vi "TalonFXConfigurator.vi"(6 "timeoutSeconds":dbl=0.05, 8 "error in":errorcluster, 10 "DeviceConfiguration":T2={"Future Proof Configs"=FALSE, "MotorOutputInverted"=0, "MotorOutputNeutralMode"=0, "MotorOutputDutyCycleNeutralDeadband"=0.0, "MotorOutputPeakForwardDutyCycle"=1.0, "MotorOutputPeakReverseDutyCycle"=-1.0, "CurrentLimitsStatorCurrentLimit"=0.0, "CurrentLimitsStatorCurrentLimitEnable"=FALSE, "CurrentLimitsSupplyCurrentLimit"=0.0, "CurrentLimitsSupplyCurrentLimitEnable"=FALSE, "CurrentLimitsSupplyCurrentThreshold"=0.0, "CurrentLimitsSupplyTimeThreshold"=0.0, "VoltageSupplyVoltageTimeConstant"=0.0, "VoltagePeakForwardVoltage"=16.0, "VoltagePeakReverseVoltage"=-16.0, "TorqueCurrentPeakForwardTorqueCurrent"=800.0, "TorqueCurrentPeakReverseTorqueCurrent"=-800.0, "TorqueCurrentTorqueNeutralDeadband"=0.0, "FeedbackFeedbackRotorOffset"=0.0, "FeedbackSensorToMechanismRatio"=1.0, "FeedbackRotorToSensorRatio"=1.0, "FeedbackFeedbackSensorSource"=0, "FeedbackFeedbackRemoteSensorID"=0, "DifferentialSensorsDifferentialSensorSource"=0, "DifferentialSensorsDifferentialTalonFXSensorID"=0, "DifferentialSensorsDifferentialRemoteSensorID"=0, "DifferentialConstantsPeakDifferentialDutyCycle"=2.0, "DifferentialConstantsPeakDifferentialVoltage"=32.0, "DifferentialConstantsPeakDifferentialTorqueCurrent"=1600.0, "OpenLoopRampsDutyCycleOpenLoopRampPeriod"=0.0, "OpenLoopRampsVoltageOpenLoopRampPeriod"=0.0, "OpenLoopRampsTorqueOpenLoopRampPeriod"=0.0, "ClosedLoopRampsDutyCycleClosedLoopRampPeriod"=0.0, "ClosedLoopRampsVoltageClosedLoopRampPeriod"=0.0, "ClosedLoopRampsTorqueClosedLoopRampPeriod"=0.0, "HardwareLimitSwitchForwardLimitType"=0, "HardwareLimitSwitchForwardLimitAutosetPositionEnable"=FALSE, "HardwareLimitSwitchForwardLimitAutosetPositionValue"=0.0, "HardwareLimitSwitchForwardLimitEnable"=TRUE, "HardwareLimitSwitchForwardLimitSource"=0, "HardwareLimitSwitchForwardLimitRemoteSensorID"=0, "HardwareLimitSwitchReverseLimitType"=0, "HardwareLimitSwitchReverseLimitAutosetPositionEnable"=FALSE, "HardwareLimitSwitchReverseLimitAutosetPositionValue"=0.0, "HardwareLimitSwitchReverseLimitEnable"=TRUE, "HardwareLimitSwitchReverseLimitSource"=0, "HardwareLimitSwitchReverseLimitRemoteSensorID"=0, "AudioBeepOnBoot"=TRUE, "AudioBeepOnConfig"=TRUE, "AudioAllowMusicDurDisable"=FALSE, "SoftwareLimitSwitchForwardSoftLimitEnable"=FALSE, "SoftwareLimitSwitchReverseSoftLimitEnable"=FALSE, "SoftwareLimitSwitchForwardSoftLimitThreshold"=0.0, "SoftwareLimitSwitchReverseSoftLimitThreshold"=0.0, "MotionMagicMotionMagicCruiseVelocity"=0.0, "MotionMagicMotionMagicAcceleration"=0.0, "MotionMagicMotionMagicJerk"=0.0, "MotionMagicMotionMagicExpo_kV"=0.0, "MotionMagicMotionMagicExpo_kA"=0.0, "CustomParamsCustomParam0"=0, "CustomParamsCustomParam1"=0, "ClosedLoopGeneralContinuousWrap"=FALSE, "Slot0kP"=0.0, "Slot0kI"=0.0, "Slot0kD"=0.0, "Slot0kS"=0.0, "Slot0kV"=0.0, "Slot0kA"=0.0, "Slot0kG"=0.0, "Slot0GravityType"=0, "Slot0StaticFeedforwardSign"=0, "Slot1kP"=0.0, "Slot1kI"=0.0, "Slot1kD"=0.0, "Slot1kS"=0.0, "Slot1kV"=0.0, "Slot1kA"=0.0, "Slot1kG"=0.0, "Slot1GravityType"=0, "Slot1StaticFeedforwardSign"=0, "Slot2kP"=0.0, "Slot2kI"=0.0, "Slot2kD"=0.0, "Slot2kS"=0.0, "Slot2kV"=0.0, "Slot2kA"=0.0, "Slot2kG"=0.0, "Slot2GravityType"=0, "Slot2StaticFeedforwardSign"=0} {"MotorOutputInverted" items=["CounterClockwise_Positive", "Clockwise_Positive"]; "MotorOutputNeutralMode" items=["Coast", "Brake"]; "FeedbackFeedbackSensorSource" items=["RotorSensor", "RemoteCANcoder", "RemotePigeon2_Yaw", "RemotePigeon2_Pitch", "RemotePigeon2_Roll", "FusedCANcoder", "SyncCANcoder"]; "DifferentialSensorsDifferentialSensorSource" items=["Disabled", "RemoteTalonFX_Diff", "RemotePigeon2_Yaw", "RemotePigeon2_Pitch", "RemotePigeon2_Roll", "RemoteCANcoder"]; "HardwareLimitSwitchForwardLimitType" items=["NormallyOpen", "NormallyClosed"]; "HardwareLimitSwitchForwardLimitSource" items=["LimitSwitchPin"=0, "RemoteTalonFX"=1, "RemoteCANifier"=2, "RemoteCANcoder"=4, "Disabled"=3]; "HardwareLimitSwitchReverseLimitType" items=["NormallyOpen", "NormallyClosed"]; "HardwareLimitSwitchReverseLimitSource" items=["LimitSwitchPin"=0, "RemoteTalonFX"=1, "RemoteCANifier"=2, "RemoteCANcoder"=4, "Disabled"=3]; "Slot0GravityType" items=["Elevator_Static", "Arm_Cosine"]; "Slot0StaticFeedforwardSign" items=["UseVelocitySign", "UseClosedLoopSign"]; "Slot1GravityType" items=["Elevator_Static", "Arm_Cosine"]; "Slot1StaticFeedforwardSign" items=["UseVelocitySign", "UseClosedLoopSign"]; "Slot2GravityType" items=["Elevator_Static", "Arm_Cosine"]; "Slot2StaticFeedforwardSign" items=["UseVelocitySign", "UseClosedLoopSign"]}, 11 "DeviceReference":T1) -> (0 "error out":errorcluster)   [LabVIEW 2023]
uses:
  Users/Cory/Documents/PhoenixPro-LabVIEW-Generation/controls/DeviceReference.ctl
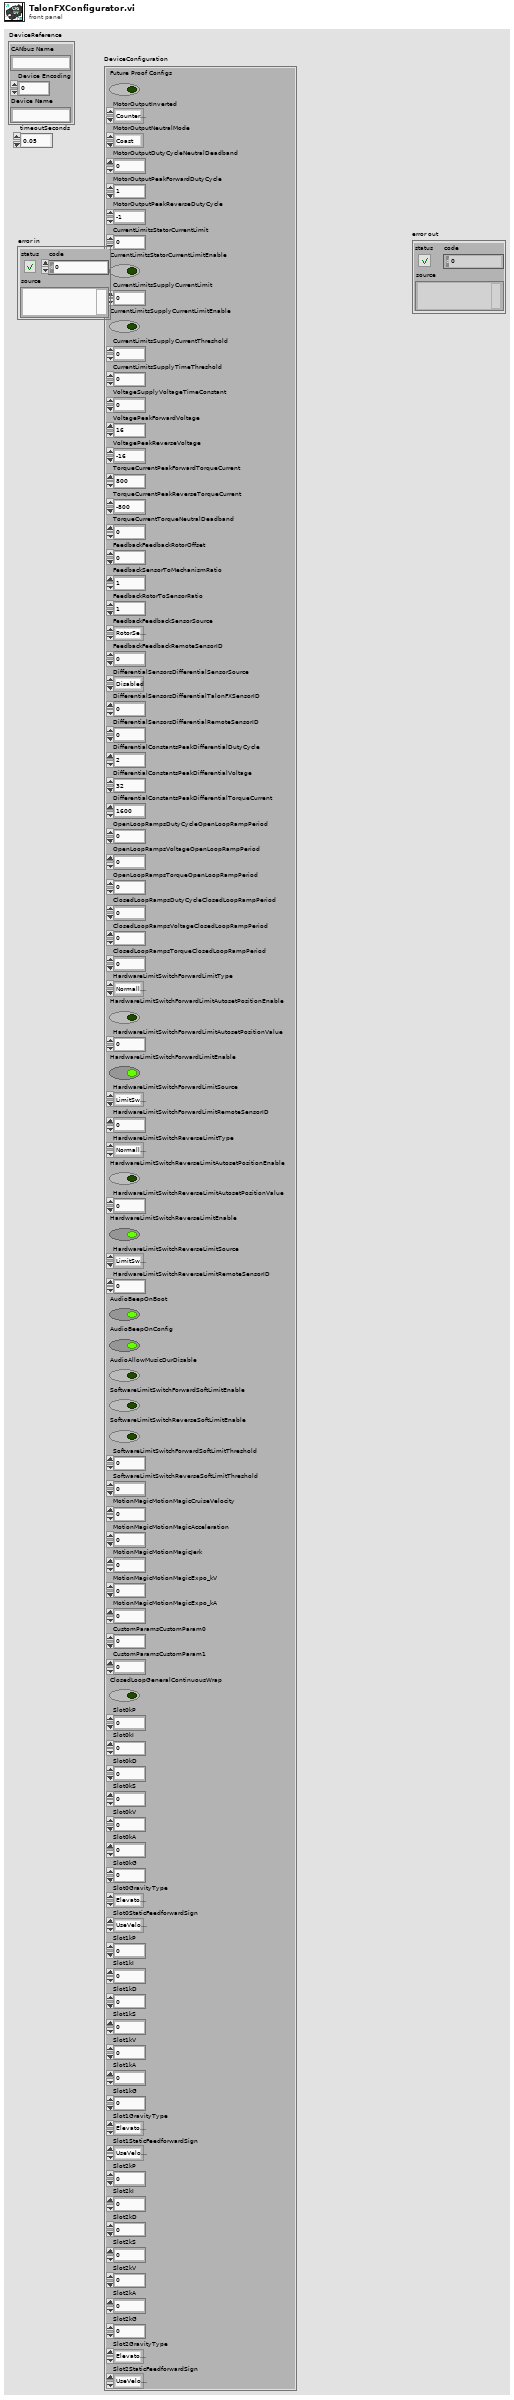
[diagram p1: front panel]
types:
  T1 = typedef "DeviceReference.ctl" = cluster{"CANbus Name":string, "Device Encoding":u32, "Device Name":string}
  T2 = cluster{"Future Proof Configs":bool, "MotorOutputInverted":u16, "MotorOutputNeutralMode":u16, "MotorOutputDutyCycleNeutralDeadband":dbl, "MotorOutputPeakForwardDutyCycle":dbl, "MotorOutputPeakReverseDutyCycle":dbl, "CurrentLimitsStatorCurrentLimit":dbl, "CurrentLimitsStatorCurrentLimitEnable":bool, "CurrentLimitsSupplyCurrentLimit":dbl, "CurrentLimitsSupplyCurrentLimitEnable":bool, "CurrentLimitsSupplyCurrentThreshold":dbl, "CurrentLimitsSupplyTimeThreshold":dbl, "VoltageSupplyVoltageTimeConstant":dbl, "VoltagePeakForwardVoltage":dbl, "VoltagePeakReverseVoltage":dbl, "TorqueCurrentPeakForwardTorqueCurrent":dbl, "TorqueCurrentPeakReverseTorqueCurrent":dbl, "TorqueCurrentTorqueNeutralDeadband":dbl, "FeedbackFeedbackRotorOffset":dbl, "FeedbackSensorToMechanismRatio":dbl, "FeedbackRotorToSensorRatio":dbl, "FeedbackFeedbackSensorSource":u16, "FeedbackFeedbackRemoteSensorID":i16, "DifferentialSensorsDifferentialSensorSource":u16, "DifferentialSensorsDifferentialTalonFXSensorID":i16, "DifferentialSensorsDifferentialRemoteSensorID":i16, "DifferentialConstantsPeakDifferentialDutyCycle":dbl, "DifferentialConstantsPeakDifferentialVoltage":dbl, "DifferentialConstantsPeakDifferentialTorqueCurrent":dbl, "OpenLoopRampsDutyCycleOpenLoopRampPeriod":dbl, "OpenLoopRampsVoltageOpenLoopRampPeriod":dbl, "OpenLoopRampsTorqueOpenLoopRampPeriod":dbl, "ClosedLoopRampsDutyCycleClosedLoopRampPeriod":dbl, "ClosedLoopRampsVoltageClosedLoopRampPeriod":dbl, "ClosedLoopRampsTorqueClosedLoopRampPeriod":dbl, "HardwareLimitSwitchForwardLimitType":u16, "HardwareLimitSwitchForwardLimitAutosetPositionEnable":bool, "HardwareLimitSwitchForwardLimitAutosetPositionValue":dbl, "HardwareLimitSwitchForwardLimitEnable":bool, "HardwareLimitSwitchForwardLimitSource":u16, "HardwareLimitSwitchForwardLimitRemoteSensorID":i16, "HardwareLimitSwitchReverseLimitType":u16, "HardwareLimitSwitchReverseLimitAutosetPositionEnable":bool, "HardwareLimitSwitchReverseLimitAutosetPositionValue":dbl, "HardwareLimitSwitchReverseLimitEnable":bool, "HardwareLimitSwitchReverseLimitSource":u16, "HardwareLimitSwitchReverseLimitRemoteSensorID":i16, "AudioBeepOnBoot":bool, "AudioBeepOnConfig":bool, "AudioAllowMusicDurDisable":bool, "SoftwareLimitSwitchForwardSoftLimitEnable":bool, "SoftwareLimitSwitchReverseSoftLimitEnable":bool, "SoftwareLimitSwitchForwardSoftLimitThreshold":dbl, "SoftwareLimitSwitchReverseSoftLimitThreshold":dbl, "MotionMagicMotionMagicCruiseVelocity":dbl, "MotionMagicMotionMagicAcceleration":dbl, "MotionMagicMotionMagicJerk":dbl, "MotionMagicMotionMagicExpo_kV":dbl, "MotionMagicMotionMagicExpo_kA":dbl, "CustomParamsCustomParam0":i16, "CustomParamsCustomParam1":i16, "ClosedLoopGeneralContinuousWrap":bool, "Slot0kP":dbl, "Slot0kI":dbl, "Slot0kD":dbl, "Slot0kS":dbl, "Slot0kV":dbl, "Slot0kA":dbl, "Slot0kG":dbl, "Slot0GravityType":u16, "Slot0StaticFeedforwardSign":u16, "Slot1kP":dbl, "Slot1kI":dbl, "Slot1kD":dbl, "Slot1kS":dbl, "Slot1kV":dbl, "Slot1kA":dbl, "Slot1kG":dbl, "Slot1GravityType":u16, "Slot1StaticFeedforwardSign":u16, "Slot2kP":dbl, "Slot2kI":dbl, "Slot2kD":dbl, "Slot2kS":dbl, "Slot2kV":dbl, "Slot2kA":dbl, "Slot2kG":dbl, "Slot2GravityType":u16, "Slot2StaticFeedforwardSign":u16}
  T3 = typedef "LVNumericRepresentation.ctl" = enum32{"Extended Precision", "Double Precision", "Single Precision", "Long", "Word", "Byte", "Unsigned Long", "Unsigned Word", "Unsigned Byte", "Complex Extended", "Complex Double", "Complex Single", "Quad", "Unsigned Quad", "Fixed-Point"}
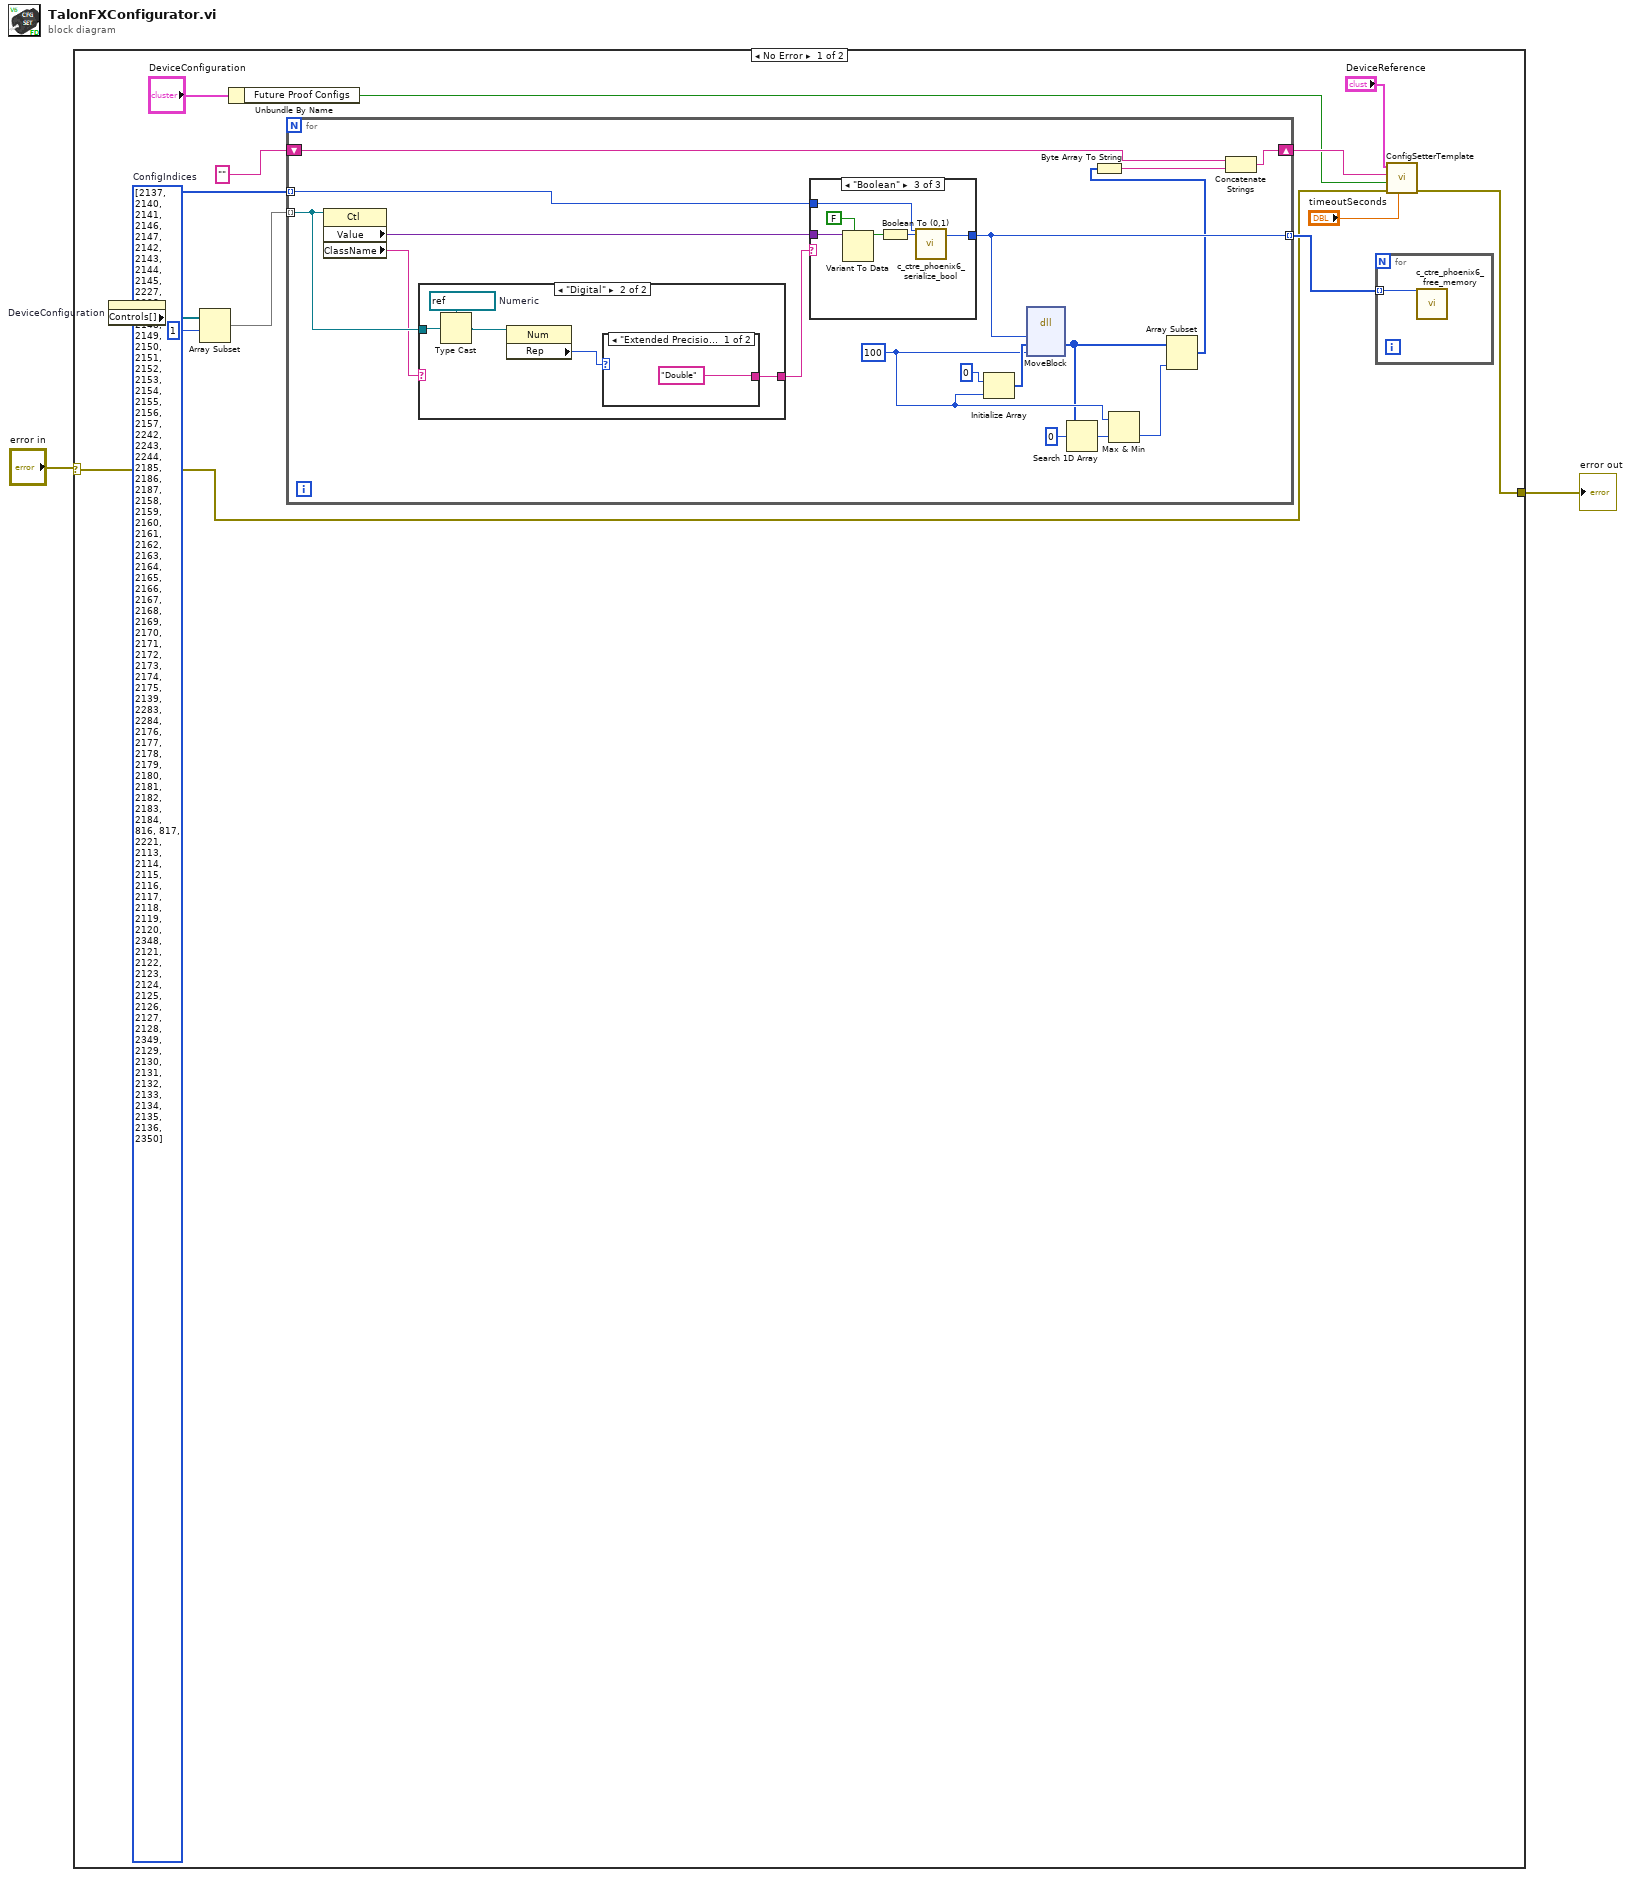
[diagram p0: block diagram]
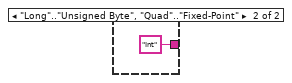
[diagram p3: hidden frame]
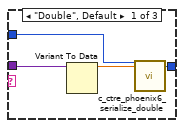
[diagram p4: hidden frame]
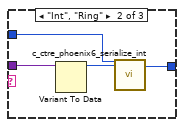
[diagram p5: hidden frame]
diagram:
  n1 = case shown="No Error" "error in" {
    selector: "error in" -> [w4 w56]
    tunnel: [w3 w56] -> w1
    frame No Error {
      w6 = i32[] [2137, 2140, 2141, 2146, 2147, 2142, 2143, 2144, 2145, 2227, 2228, 2138, 2148, 2149, 2150, 2151, 2152, 2153, 2154, 2155, 2156, 2157, 2242, 2243, 2244, 2185, 2186, 2187, 2158, 2159, 2160, 2161, 2162, 2163, 2164, 2165, 2166, 2167, 2168, 2169, 2170, 2171, 2172, 2173, 2174, 2175, 2139, 2283, 2284, 2176, 2177, 2178, 2179, 2180, 2181, 2182, 2183, 2184, 816, 817, 2221, 2113, 2114, 2115, 2116, 2117, 2118, 2119, 2120, 2348, 2121, 2122, 2123, 2124, 2125, 2126, 2127, 2128, 2349, 2129, 2130, 2131, 2132, 2133, 2134, 2135, 2136, 2350]  # ConfigIndices
      n2 = property on="DeviceConfiguration" class="Clust (strict)"() -> ("Controls[]"=w9:refnum<vi>[])  [unwired: 2 in, 2 out]
      n3 = Array Subset(array=w9, index=1) -> (w10:refnum<vi>[])  [unwired: 1 in]
      n4 = Unbundle By Name("DeviceConfiguration") -> ("Future Proof Configs"=w5:bool)
      n5 = for {
        tunnel: w10 -> [w27] mode=indexing
        shift-right: [w30] -> w14
        shift-left: "" -> [w31]
        tunnel: [w22] -> w7 mode=indexing
        tunnel: w6 -> [w28] mode=indexing
        w18 = i64 100 ("size")
        n6 = property class="Ctl"(reference=w27) -> ("Value"=w32:variant, "ClassName"=w26:string)  [unwired: 1 in, 2 out]
        n7 = case shown="\"Digital\"" w26 {
          selector: w26 -> [w33 _]
          tunnel: w27 -> [_ w36]
          tunnel: [w33 w37] -> w25
          frame Default {
          }
          frame "Digital" {
            w34 = refnum<vi> refnum  # Numeric
            n8 = Type Cast(type=w34, x=w36) -> (*(type *) &x=w35:refnum<vi>)
            n9 = property class="Num"(reference=w35) -> ("Rep"=w38:T3)  [unwired: 1 in, 2 out]
            n10 = case shown="\"Extended Precision\"..\"Single Precision\", \"Complex Extended\"..\"Complex Single\"" w38 {
              tunnel: ["Double" "Int"] -> w37
              frame "Extended Precision".."Single Precision", "Complex Extended".."Complex Single" {
              }
              frame "Long".."Unsigned Byte", "Quad".."Fixed-Point" {
              }
            }
          }
        }
        n11 = case shown="\"Boolean\"" w25 {
          tunnel: w32 -> [w42 w48 w54]
          tunnel: [w43 w46 w53] -> w22
          tunnel: w28 -> [w41 w45 w52]
          frame "Double", Default {
            n12 = Variant To Data(Variant=w42) -> (data=w44:dbl)  [unwired: 2 in, 1 out]
            n13 = call <vilib>:"c_ctre_phoenix6_serialize_double.vi"("Numeric 2"=w41, "Numeric 3"=w44) -> ("Numeric 4"=w43:u32)  [unwired: 24 in, 1 out]
          }
          frame "Int", "Ring" {
            n14 = Variant To Data(Variant=w48) -> (data=w47:i32)  [unwired: 2 in, 1 out]
            n15 = call <vilib>:"c_ctre_phoenix6_serialize_int.vi"("Numeric 2"=w45, "Numeric 3"=w47) -> ("Numeric 4"=w46:u32)  [unwired: 24 in, 1 out]
          }
          frame "Boolean" {
            n16 = Variant To Data(type=FALSE, Variant=w54) -> (data=w50:bool)  [unwired: 1 in, 1 out]
            n17 = Boolean To (0,1)(Boolean=w50) -> (0, 1=w49:i16)
            n18 = call <vilib>:"c_ctre_phoenix6_serialize_bool.vi"("Numeric 2"=w52, "Numeric 3"=w49) -> ("Numeric 4"=w53:u32)  [unwired: 24 in, 1 out]
          }
        }
        n19 = Initialize Array(u8 0 ("element"), w18) -> (w24:u8[])
        n20 = dll-call lib="LabVIEW" fn="MoveBlock"("ps"=w22, "pd"=w24, "size"=w18) -> ("pd"=w17:u8[])  [unwired: 6 in, 2 out]
        n21 = Search 1D Array(1D array=w17, element=u8 0) -> (index of element=w19:i32)  [unwired: 1 in]
        n22 = Max & Min(x=w18, y=w19) -> (min(x,y)=w16:i64)  [unwired: 1 out]
        n23 = Array Subset(array=w17, length=w16) -> (w21:u8[])  [unwired: 1 in]
        n24 = Byte Array To String(unsigned byte array=w21) -> (string=w29:string)
        n25 = Concatenate Strings(w31, w29) -> (w30:string)
      }
      n26 = for {
        tunnel: w7 -> [w55] mode=indexing
        n27 = call <vilib>:"c_ctre_phoenix6_free_memory.vi"("Numeric 3"=w55) -> ()  [unwired: 25 in, 2 out]
      }
      n28 = call "ConfigSetterTemplate.vi"("timeoutSeconds"="timeoutSeconds", "error in"=w4, "FutureProofConfigs"=w5, "Configs"=w14, "DeviceReference"="DeviceReference") -> ("error out"=w3:errorcluster)  [unwired: 6 in]
    }
    frame Error {
    }
  }
  "error out" <- w1
